vi "Preset terminal map id.vi"(2 "Terminal Data in":T1[](array[typedef]) {"Terminal Flags" format="%.0b"}) -> (0 "Terminal Data out":T1[](array[typedef]) {"Terminal Flags" format="%.0b"})   [LabVIEW 2020, in "GetSetShared.lvlib"]
uses:
  <vilib>/express/express signal manip/GetorSetDDTAttributes/Shared VIs/GetSetShared.lvlib
  <vilib>/BlockNodeSupport/TerminalData.ctl
  <vilib>/express/express signal manip/GetorSetDDTAttributes/Shared VIs/Global 1.vi
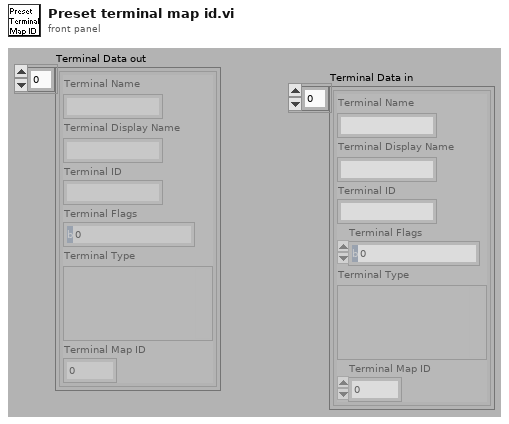
[diagram p1: front panel]
types:
  T1 = typedef "TerminalData.ctl" = cluster{"Terminal Name":string, "Terminal Display Name":string, "Terminal ID":string, "Terminal Flags":i32, "Terminal Type":variant, "Terminal Map ID":i32}
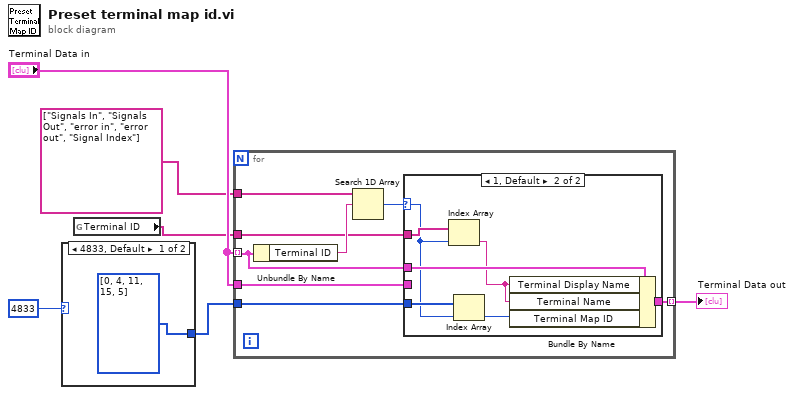
[diagram p0: block diagram]
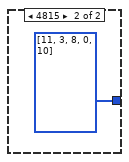
[diagram p2: hidden frame]
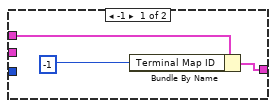
[diagram p3: hidden frame]
diagram:
  n1 = case shown="4833, Default" 4833 ("CP Type") {
    tunnel: [i32[] [0, 4, 11, 15, 5] ("Terminal Map ID") i32[] [11, 3, 8, 0, 10] ("Terminal Map ID")] -> w4
    frame 4833, Default {
    }
    frame 4815 {
    }
  }
  n2 = global read "Global 1.vi" "Terminal ID"() -> (w1:string[])
  n3 = for {
    tunnel: "Terminal Data in" -> [w10] mode=indexing
    tunnel: string[] ["Signals In", "Signals Out", "error in", "error out", "Signal Index"] ("Terminal ID") -> [w16]
    tunnel: "Terminal Data in" -> [w14]
    tunnel: [w12] -> w5 mode=indexing
    tunnel: w4 -> [w13]
    tunnel: w1 -> [w9]
    n4 = Unbundle By Name(w10) -> ("Terminal ID"=w15:string)
    n5 = Search 1D Array(1D array=w16, element=w15) -> (index of element=w11:i32)  [unwired: 1 out]
    n6 = case shown="1, Default" w11 {
      selector: w11 -> [_ w21]
      tunnel: w14 -> [_ _]
      tunnel: w13 -> [_ w26]
      tunnel: [w17 w25] -> w12
      tunnel: w10 -> [w19 w23]
      tunnel: w9 -> [_ w22]
      frame -1 {
        n7 = Bundle By Name(cluster=w19, "Terminal Map ID"=-1) -> (w17:T1)
      }
      frame 1, Default {
        n8 = Index Array(array=w22, index=w21) -> (element=w20:string)
        n9 = Index Array(array=w26, index=w21) -> (element=w24:i32)
        n10 = Bundle By Name(cluster=w23, "Terminal Display Name"=w20, "Terminal Name"=w20, "Terminal Map ID"=w24) -> (w25:T1)
      }
    }
  }
  "Terminal Data out" <- w5
